vi "utm_midpoint.vi"(10 "UTM Location 2":T1 {"North" format="%#_10f"; "East" format="%#_8f"}, 11 "UTM Location":T1 {"North" format="%#_10f"; "East" format="%#_8f"}) -> (1 "Distance from given to intermediate point":dbl, 2 "Distance between given points":dbl, 3 "UTM Location 3":T1 {"North" format="%#_10f"; "East" format="%#_8f"})   [LabVIEW 2013]
doc: "Finds the midpoint between two UTM coordinates and returns it in UTM.\n\nDoes not take into account UTM zones or hemispheres."
uses:
  Data/TypeDefs/UTM Location.ctl
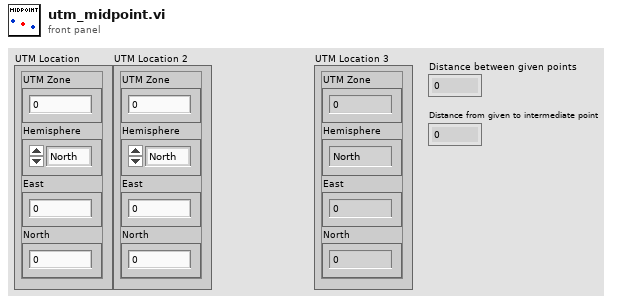
[diagram p1: front panel]
types:
  T1 = typedef "UTM Location.ctl" = cluster{"UTM Zone":dbl, "Hemisphere":enum16{"North", "South"}, "East":dbl, "North":dbl}
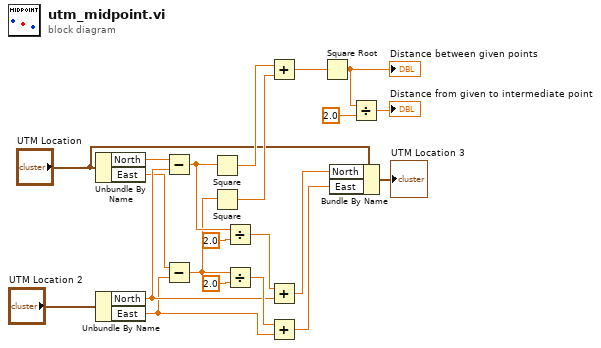
[diagram p0: block diagram]
diagram:
  n1 = Unbundle By Name("UTM Location") -> ("North"=w13:dbl, "East"=w12:dbl)
  n2 = Unbundle By Name("UTM Location 2") -> ("North"=w17:dbl, "East"=w16:dbl)
  n3 = Subtract(x=w13, y=w17) -> (x-y=w8:dbl)
  n4 = Subtract(x=w12, y=w16) -> (x-y=w7:dbl)
  n5 = Square(x=w8) -> (x^2=w10:dbl)
  n6 = Square(x=w7) -> (x^2=w11:dbl)
  n7 = Divide(x=w8, y=2.0) -> (x/y=w18:dbl)
  n8 = Divide(x=w7, y=2.0) -> (x/y=w19:dbl)
  n9 = Add(x=w10, y=w11) -> (x+y=w9:dbl)
  n10 = Add(x=w18, y=w17) -> (x+y=w14:dbl)
  n11 = Add(x=w19, y=w16) -> (x+y=w15:dbl)
  n12 = Square Root(x=w9) -> (sqrt(x)=w3:dbl)
  "Distance between given points" <- w3
  n13 = Bundle By Name(cluster="UTM Location", "North"=w14, "East"=w15) -> (→"UTM Location 3":T1)
  n14 = Divide(x=w3, y=2.0) -> (x/y=→"Distance from given to intermediate point":dbl)
